vi "RP Write Command.vi"(7 "Config offset":u64 format="%x", 8 "Error In":errorcluster, 9 "Command payload":u64 format="%x", 10 "Command number":T1, 11 "connection ID":refnum<k5>) -> (0 "Error Out":errorcluster, 2 "bytes written":i32, 3 "connection ID out":refnum<k5>)   [LabVIEW 2015]
uses:
  RP Command.ctl
panel:
  out "x .or. y?":u64 format="%x"
  out "x << y":u64 format="%x"
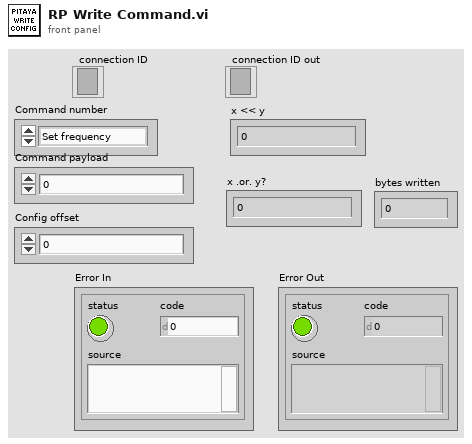
[diagram p1: front panel]
types:
  T1 = typedef "RP Command.ctl" = enum16{"Set frequency", "Arm and get data", "Stop server", "Get status", "Get temperature", "Set decimation", "Arm", "Software trigger", "Get whole buffer", "Get chunk", "System call", "Get config", "Set config", "Read FIFO", "Play pattern", "Set frequency batch"}
  T2 = enum16{"big-endian, network order", "native, host order", "little-endian"}
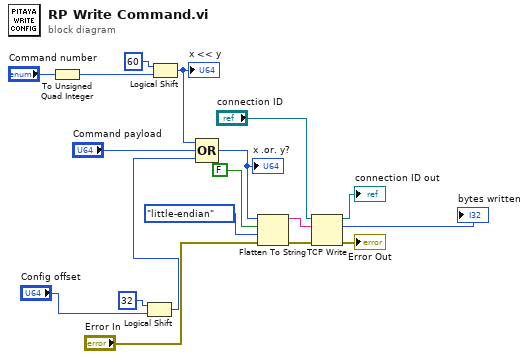
[diagram p0: block diagram]
diagram:
  n1 = To Unsigned Quad Integer(1:"Command number") -> (0:w4:u64)
  n2 = Logical Shift(y=i16 32, x="Config offset") -> (x << y=w1:u64)
  n3 = Logical Shift(y=i16 60, x=w4) -> (x << y=w16:u64)
  "x << y" <- w16
  n4 = Compound Arithmetic op=OR(w16, "Command payload", w1) -> (w6:u64)
  "x .or. y?" <- w6
  n5 = Flatten To String(anything=w6, prepend array or string size? (T)=FALSE, byte order (0:big-endian, network order)=T2."little-endian", error in (no error)="Error In") -> (data string=w10:string, error out=w11:errorcluster)  [unwired: 1 out]
  n6 = TCP Write(connection ID="connection ID", data in=w10, error in (no error)=w11) -> (connection ID out=→"connection ID out":refnum<k5>, bytes written=→"bytes written":i32, error out=→"Error Out":errorcluster)  [unwired: 1 in]
